vi "Perform Mem Test.vi"(8 "error in (no error)":errorcluster, 11 "LCM Single-Up MTS Test in":refnum<class "LCM Single-Up MTS Test.lvclass">) -> (0 "error out":errorcluster, 3 "Memory Test Passed":bool)   [LabVIEW 2015, in "LCM Single-Up MTS Test.lvclass"]
uses:
  LCM Single-Up MTS Test.lvclass
  <vilib>/Cree, Inc/Cree Test Framework/Core Launcher/Core Manager Methods -- Enum.ctl
  <vilib>/Cree, Inc/Cree Test Framework/Core Launcher/Core Launcher.lvlib
  <vilib>/Cree, Inc/Cree Test Framework/Classes/Data/Data Repo/Class/Data Repo.lvclass
  Classes/Manufacturing Test/Class/SC Manufacturing Test.lvclass
  <vilib>/Cree, Inc/Cree Test Framework/Classes/Base Objects/Base Class/Base Class/Base Class.lvclass
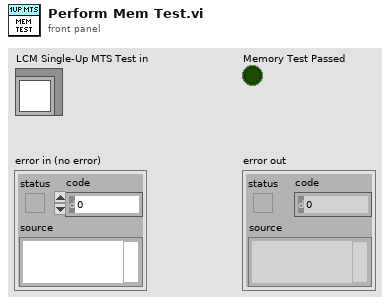
[diagram p1: front panel]
types:
  T1 = typedef "Core Launcher.lvlib/Core Manager Methods -- Enum.ctl" = enum16{"Spawn Objects", "Get Objects", "Destroy Objects"}
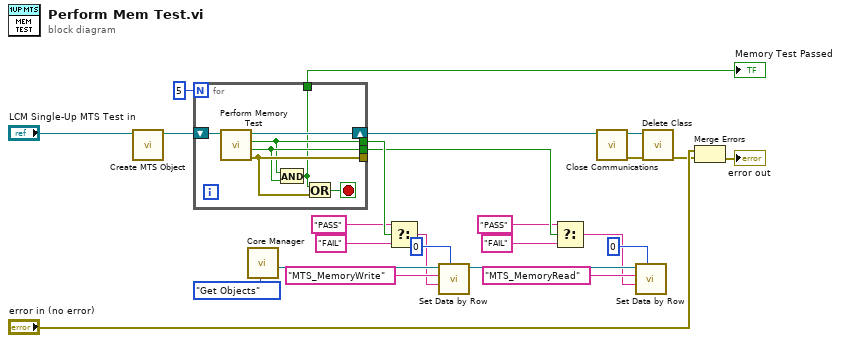
[diagram p0: block diagram]
diagram:
  n1 = call "Create MTS Object.vi"("LCM Single-Up MTS Test in"="LCM Single-Up MTS Test in") -> ("MTS"=w6:refnum<class "SC Manufacturing Test.lvclass">)  [unwired: 9 in, 1 out]
  n2 = for {
    N: 5 -> [_]
    shift-right: [w32] -> w4
    shift-left: w6 -> [w31]
    tunnel: [w28] -> w21
    tunnel: [w27] -> w22
    tunnel: [w26] -> w5
    tunnel: [w29] -> _
    stop <- w30 stop-if-true
    n3 = call "Perform Memory Test.vi"("Acrobat Template in"=w31) -> ("error out"=w29:errorcluster, "Read Passed"=w28:bool, "Write Passed"=w27:bool, "Acrobat Template out"=w32:refnum<class "SC Manufacturing Test.lvclass">)  [unwired: 7 in]
    n4 = And(x=w27, y=w28) -> (x .and. y?=w26:bool)
    n5 = Or(x=w26, y=w29) -> (x .or. y?=w30:bool)
  }
  "Memory Test Passed" <- w5
  n6 = call <vilib>:"Core Manager.vi"("Method"=Core_Manager_Methods_--_Enum."Get Objects") -> ("Data Repo"=w19:refnum<class "Data Repo.lvclass">)  [unwired: 6 in, 4 out]
  n7 = Select(t="PASS" ("Header"), s=w22, f="FAIL" ("Header")) -> (s? t:f=w14:string)
  n8 = call <vilib>:"Set Data by Row.vi"("Row"=0, "Value"=w14, "Header"="MTS_MemoryWrite", "Acrobat Template in"=w19) -> ("Acrobat Template out"=w12:refnum<class "Data Repo.lvclass">)  [unwired: 6 in, 1 out]
  n9 = Select(t="PASS" ("Header"), s=w21, f="FAIL" ("Header")) -> (s? t:f=w8:string)
  n10 = call "Close Communications.vi"("Acrobat Template in"=w4) -> ("error out"=w2:errorcluster, "Acrobat Template out"=w3:refnum<class "SC Manufacturing Test.lvclass">)  [unwired: 9 in]
  n11 = call <vilib>:"Set Data by Row.vi"("Row"=0, "Value"=w8, "Header"="MTS_MemoryRead", "Acrobat Template in"=w12) -> ()  [unwired: 6 in, 2 out]
  n12 = call <vilib>:"Delete Class.vi"("error in (no error)"=w2, "Base Class in"=w3) -> ("error out"=w1:errorcluster)  [unwired: 8 in, 1 out]
  n13 = Merge Errors("error in (no error)", w1) -> (→"error out":errorcluster)
